vi "parsePosition.vi"(8 "error in (no error)":errorcluster, 10 "position":string, 11 "AlCS in":refnum<class "AlCS.lvclass">) -> (0 "error out":errorcluster, 2 "position":T2, 3 "AlCS out":refnum<class "AlCS.lvclass">)   [LabVIEW 2016, in "AlCS.lvclass"]
uses:
  AlCS.lvclass
  Subsystems.ctl
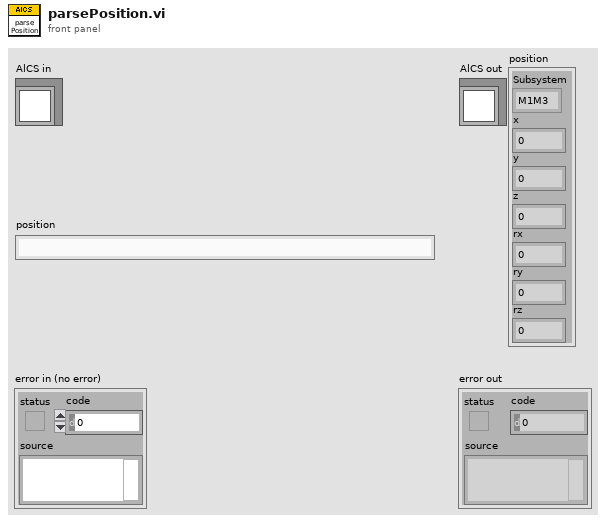
[diagram p1: front panel]
types:
  T1 = typedef "Subsystems.ctl" = enum16{"M1M3", "Camera", "M2"}
  T2 = cluster{"Subsystem":T1, "x":dbl, "y":dbl, "z":dbl, "rx":dbl, "ry":dbl, "rz":dbl}
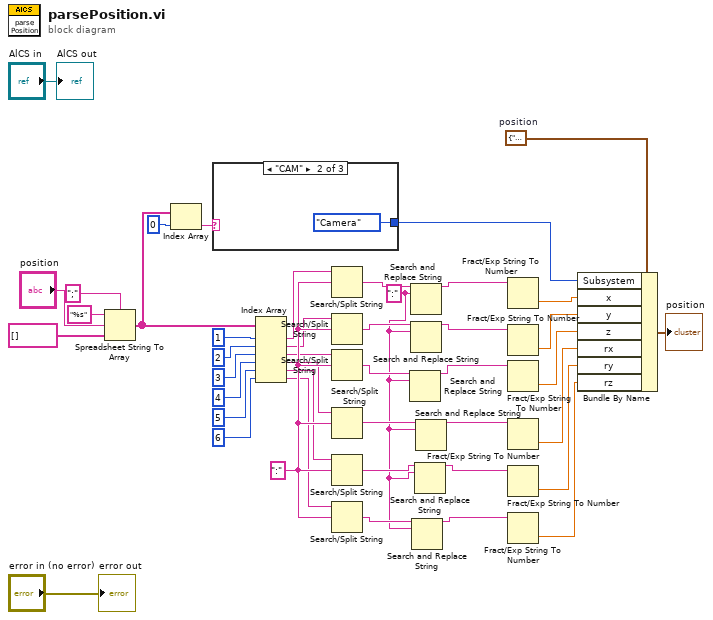
[diagram p0: block diagram]
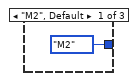
[diagram p2: hidden frame]
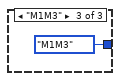
[diagram p3: hidden frame]
diagram:
  w1 = ":" ("search string")
  w27 = ":" ("search string/char (-)")
  w35 = T2 {"Subsystem"=enum."M1M3", "x"=0.0, "y"=0.0, "z"=0.0, "rx"=0.0, "ry"=0.0, "rz"=0.0}  # position
  n1 = Spreadsheet String To Array(delimiter (Tab)=";", format string="%s", spreadsheet string="position", array type (2D Dbl)=string[] []) -> (array=w36:string[])
  n2 = Index Array(array=w36, index=0) -> (element=w37:string)
  n3 = case shown="\"CAM\"" w37 {
    tunnel: [Subsystems."M2" ("Subsystem") Subsystems."Camera" ("Subsystem") Subsystems."M1M3" ("Subsystem")] -> w34
    frame "M2", Default {
    }
    frame "CAM" {
    }
    frame "M1M3" {
    }
  }
  n4 = Index Array(array=w36, index #1=1 ("index"), index #2=2 ("index"), index #3=3 ("index"), index #4=4 ("index"), index #5=5 ("index"), index #6=6 ("index")) -> (element #1=w26:string, element #2=w25:string, element #3=w24:string, element #4=w23:string, element #5=w22:string, element #6=w21:string)
  n5 = Search/Split String(string=w26, search string/char (-)=w27) -> (match + rest of string=w13:string)  [unwired: 1 in, 2 out]
  n6 = Search/Split String(string=w25, search string/char (-)=w27) -> (match + rest of string=w8:string)  [unwired: 1 in, 2 out]
  n7 = Search/Split String(string=w24, search string/char (-)=w27) -> (match + rest of string=w9:string)  [unwired: 1 in, 2 out]
  n8 = Search/Split String(string=w23, search string/char (-)=w27) -> (match + rest of string=w10:string)  [unwired: 1 in, 2 out]
  n9 = Search/Split String(string=w22, search string/char (-)=w27) -> (match + rest of string=w11:string)  [unwired: 1 in, 2 out]
  n10 = Search/Split String(string=w21, search string/char (-)=w27) -> (match + rest of string=w12:string)  [unwired: 1 in, 2 out]
  n11 = Search and Replace String(input string=w9, search string=w1) -> (result string=w5:string)  [unwired: 6 in, 3 out]
  n12 = Search and Replace String(input string=w13, search string=w1) -> (result string=w7:string)  [unwired: 6 in, 3 out]
  n13 = Search and Replace String(input string=w8, search string=w1) -> (result string=w6:string)  [unwired: 6 in, 3 out]
  n14 = Search and Replace String(input string=w12, search string=w1) -> (result string=w2:string)  [unwired: 6 in, 3 out]
  n15 = Search and Replace String(input string=w11, search string=w1) -> (result string=w3:string)  [unwired: 6 in, 3 out]
  n16 = Search and Replace String(input string=w10, search string=w1) -> (result string=w4:string)  [unwired: 6 in, 3 out]
  n17 = Fract/Exp String To Number(string=w7) -> (number=w15:dbl)  [unwired: 3 in, 1 out]
  n18 = Fract/Exp String To Number(string=w6) -> (number=w16:dbl)  [unwired: 3 in, 1 out]
  n19 = Fract/Exp String To Number(string=w5) -> (number=w17:dbl)  [unwired: 3 in, 1 out]
  n20 = Fract/Exp String To Number(string=w4) -> (number=w18:dbl)  [unwired: 3 in, 1 out]
  n21 = Fract/Exp String To Number(string=w3) -> (number=w19:dbl)  [unwired: 3 in, 1 out]
  n22 = Fract/Exp String To Number(string=w2) -> (number=w20:dbl)  [unwired: 3 in, 1 out]
  n23 = Bundle By Name(cluster=w35, "Subsystem"=w34, "x"=w15, "y"=w16, "z"=w17, "rx"=w18, "ry"=w19, "rz"=w20) -> (→"position":T2)
  "error out" <- "error in (no error)"
  "AlCS out" <- "AlCS in"
